vi "Build Design Cluster from String_2.vi"(10 "Design ID":i32, 11 "Stripe String":string) -> (3 "Stripe Data":T1)   [LabVIEW 2024]
uses:
  Cluster_Design Data_2.ctl
  ENUM_Stripe Select.ctl
  Cluster_Design Towel ID Data_2.ctl
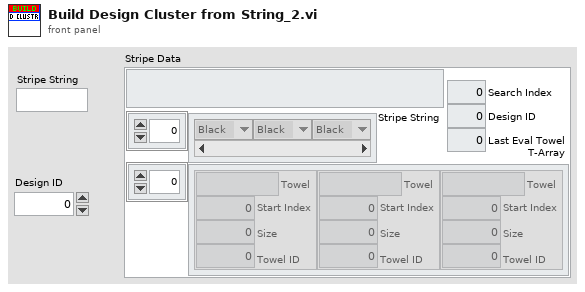
[diagram p1: front panel]
types:
  T1 = typedef "Cluster_Design Data_2.ctl" = cluster{"Stripe String":string, "Stripes":T2[], "T-Array":T3[], "Search Index":i32, "Design ID":i32, "Last Eval Towel":i32}
  T2 = typedef "ENUM_Stripe Select.ctl" = enum16{"Black", "Blue", "Green", "Red", "White"}
  T3 = typedef "Cluster_Design Towel ID Data_2.ctl" = cluster{"Towel":string, "Start Index":i32, "Size":i32, "Towel ID":i32}
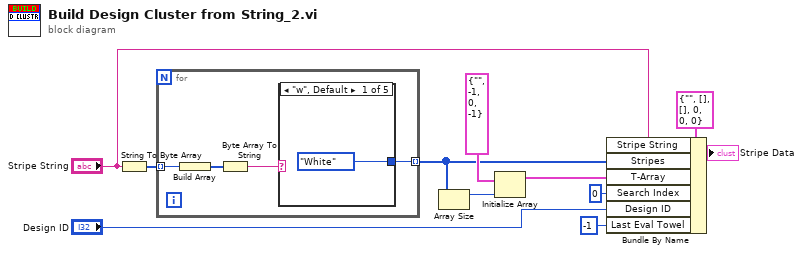
[diagram p0: block diagram]
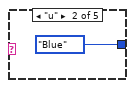
[diagram p2: hidden frame]
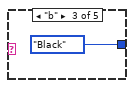
[diagram p3: hidden frame]
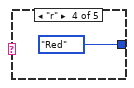
[diagram p4: hidden frame]
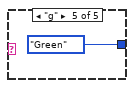
[diagram p5: hidden frame]
diagram:
  n1 = String To Byte Array(string="Stripe String") -> (unsigned byte array=w4:u8[])
  n2 = for {
    tunnel: w4 -> [w15] mode=indexing
    tunnel: [w12] -> w8 mode=indexing
    n3 = Build Array(w15) -> (w14:u8[])
    n4 = Byte Array To String(unsigned byte array=w14) -> (string=w13:string)
    n5 = case shown="\"w\", Default" w13 {
      tunnel: [ENUM_Stripe_Select."White" ("Stripe Select") ENUM_Stripe_Select."Blue" ("Stripe Select") ENUM_Stripe_Select."Black" ("Stripe Select") ENUM_Stripe_Select."Red" ("Stripe Select") ENUM_Stripe_Select."Green" ("Stripe Select")] -> w12
      frame "w", Default {
      }
      frame "u" {
      }
      frame "b" {
      }
      frame "r" {
      }
      frame "g" {
      }
    }
  }
  n6 = Array Size(array=w8) -> (size(s)=w9:i32)
  n7 = Initialize Array(T3 {"Towel"="", "Start Index"=-1, "Size"=0, "Towel ID"=-1} ("Data"), w9) -> (w11:T3[])
  n8 = Bundle By Name(cluster=T1 {"Stripe String"="", "Stripes"=[], "T-Array"=[], "Search Index"=0, "Design ID"=0, "Last Eval Towel"=0}, "Stripe String"="Stripe String", "Stripes"=w8, "T-Array"=w11, "Search Index"=0, "Design ID"="Design ID", "Last Eval Towel"=-1) -> (→"Stripe Data":T1)
